vi "Get All Classes Properties and Methods.vi"(8 "error in":errorcluster) -> (0 "error out":errorcluster, 1 "Methods[]":T1(array[cluster]), 2 "Properties[]":T2(array[cluster]), 3 "All Classes Tree Sorted":T3(array[cluster]))   [LabVIEW 2023]
doc: "Gets all classes, properties, and methods available in LabVIEW. This is slow, as it also gets the R/W-ability, if scripting, private, etc. Best to do this once and cache the results."
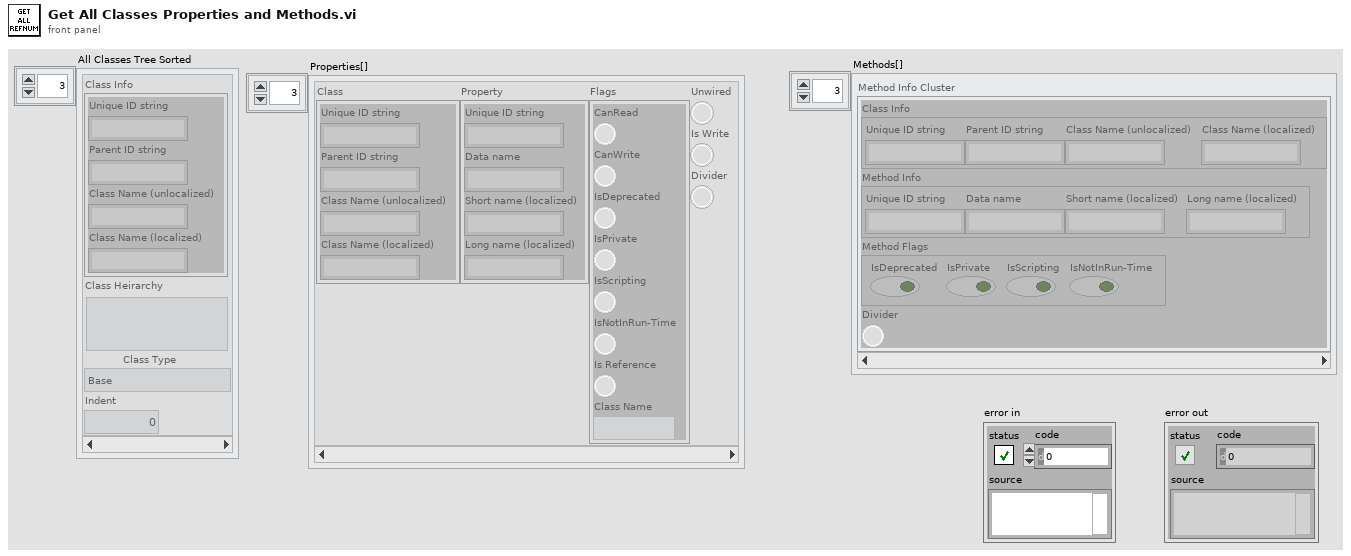
[diagram p1: front panel]
types:
  T1 = cluster{"Class Info":cluster{"Unique ID string":string, "Parent ID string":string, "Class Name (unlocalized)":string, "Class Name (localized)":string}, "Method Info":cluster{"Unique ID string":string, "Data name":string, "Short name (localized)":string, "Long name (localized)":string}, "Method Flags":cluster{"IsDeprecated":bool, "IsPrivate":bool, "IsScripting":bool, "IsNotInRun-Time":bool}, "Divider":bool}[]
  T2 = cluster{"Class":cluster{"Unique ID string":string, "Parent ID string":string, "Class Name (unlocalized)":string, "Class Name (localized)":string}, "Property":cluster{"Unique ID string":string, "Data name":string, "Short name (localized)":string, "Long name (localized)":string}, "Flags":cluster{"CanRead":bool, "CanWrite":bool, "IsDeprecated":bool, "IsPrivate":bool, "IsScripting":bool, "IsNotInRun-Time":bool, "Is Reference":bool, "Class Name":string}, "Divider":bool, "Is Write":bool, "Unwired":bool}[]
  T3 = cluster{"Class Info":cluster{"Unique ID string":string, "Parent ID string":string, "Class Name (unlocalized)":string, "Class Name (localized)":string}, "Class Heirarchy":string, "Class Type":enum16{"Unknown", "Base", "Scripting", "Private", "Deprecated", "None", "Divider"}, "Indent":u32}[]
  T4 = cluster{"Class Info":cluster{"Unique ID string":string, "Parent ID string":string, "Class Name (unlocalized)":string, "Class Name (localized)":string}, "Property Info":cluster{"Unique ID string":string, "Data name":string, "Short name (localized)":string, "Long name (localized)":string}, "Property Flags":cluster{"CanRead":bool, "CanWrite":bool, "IsDeprecated":bool, "IsPrivate":bool, "IsScripting":bool, "IsNotInRun-Time":bool, "Is Reference":bool, "Class Name":string}}[]
  T5 = cluster{"Class":cluster{"Unique ID string":string, "Parent ID string":string, "Class Name (unlocalized)":string, "Class Name (localized)":string}, "Property":cluster{"Unique ID string":string, "Data name":string, "Short name (localized)":string, "Long name (localized)":string}, "Flags":cluster{"CanRead":bool, "CanWrite":bool, "IsDeprecated":bool, "IsPrivate":bool, "IsScripting":bool, "IsNotInRun-Time":bool, "Is Reference":bool, "Class Name":string}, "Divider":bool, "Is Write":bool, "Unwired":bool}
  T6 = cluster{"Unique ID string":string, "Parent ID string":string, "Class Name (unlocalized)":string, "Class Name (localized)":string}
  T7 = cluster{"Unique ID string":string, "Data name":string, "Short name (localized)":string, "Long name (localized)":string}
  T8 = cluster{"CanRead":bool, "CanWrite":bool, "IsDeprecated":bool, "IsPrivate":bool, "IsScripting":bool, "IsNotInRun-Time":bool, "Is Reference":bool, "Class Name":string}
  T9 = cluster{"Class Info":cluster{"Unique ID string":string, "Parent ID string":string, "Class Name (unlocalized)":string, "Class Name (localized)":string}, "Method Info":cluster{"Unique ID string":string, "Data name":string, "Short name (localized)":string, "Long name (localized)":string}, "Method Flags":cluster{"IsDeprecated":bool, "IsPrivate":bool, "IsScripting":bool, "IsNotInRun-Time":bool}}[]
  T10 = cluster{"Class Info":cluster{"Unique ID string":string, "Parent ID string":string, "Class Name (unlocalized)":string, "Class Name (localized)":string}, "Method Info":cluster{"Unique ID string":string, "Data name":string, "Short name (localized)":string, "Long name (localized)":string}, "Method Flags":cluster{"IsDeprecated":bool, "IsPrivate":bool, "IsScripting":bool, "IsNotInRun-Time":bool}, "Divider":bool}
  T11 = cluster{"IsDeprecated":bool, "IsPrivate":bool, "IsScripting":bool, "IsNotInRun-Time":bool}
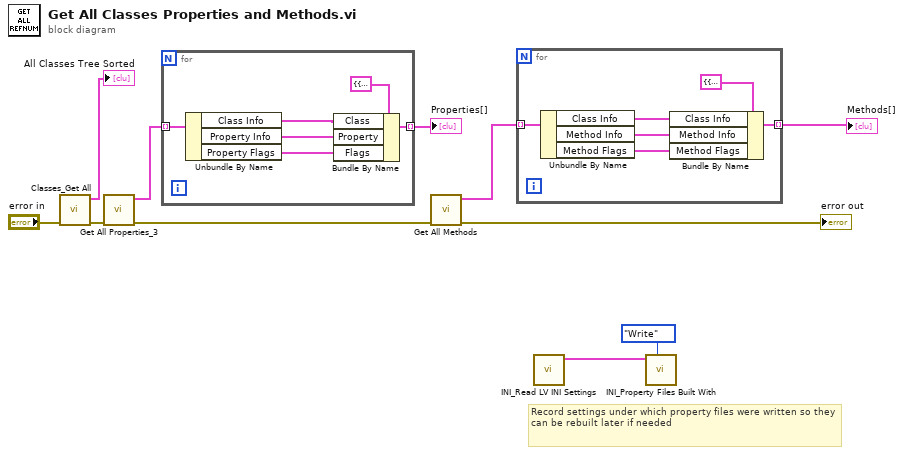
[diagram p0: block diagram]
diagram:
  # "Record settings under which property files were written so they can be rebuilt later if needed"
  n1 = call "Classes_Get All.vi"("error in"="error in") -> ("error out"=w10:errorcluster, "All Classes Tree Sorted"=→"All Classes Tree Sorted":T3)  [unwired: 9 in]
  n2 = call "Get All Properties_3.vi"("error in"=w10) -> ("error out"=w9:errorcluster, "Properties[]"=w5:T4)  [unwired: 9 in]
  n3 = for {
    tunnel: [w17] -> w6 mode=indexing
    tunnel: w5 -> [w15] mode=indexing
    n4 = Unbundle By Name(w15) -> ("Class Info"=w14:T6, "Property Info"=w13:T7, "Property Flags"=w12:T8)
    n5 = Bundle By Name(cluster=T5 {"Class"={"Unique ID string"="", "Parent ID string"="", "Class Name (unlocalized)"="", "Class Name (localized)"=""}, "Property"={"Unique ID string"="", "Data name"="", "Short name (localized)"="", "Long name (localized)"=""}, "Flags"={"CanRead"=FALSE, "CanWrite"=FALSE, "IsDeprecated"=FALSE, "IsPrivate"=FALSE, "IsScripting"=FALSE, "IsNotInRun-Time"=FALSE, "Is Reference"=FALSE, "Class Name"=""}, "Divider"=FALSE, "Is Write"=FALSE, "Unwired"=FALSE} ("Cluster"), "Class"=w14, "Property"=w13, "Flags"=w12) -> (w17:T5)
  }
  "Properties[]" <- w6
  n6 = call "Get All Methods.vi"("error in (no error)"=w9) -> ("error out"=→"error out":errorcluster, "Methods[]"=w4:T9)  [unwired: 9 in]
  n7 = for {
    tunnel: [w23] -> w3 mode=indexing
    tunnel: w4 -> [w21] mode=indexing
    n8 = Unbundle By Name(w21) -> ("Class Info"=w20:T6, "Method Info"=w19:T7, "Method Flags"=w18:T11)
    n9 = Bundle By Name(cluster=T10 {"Class Info"={"Unique ID string"="", "Parent ID string"="", "Class Name (unlocalized)"="", "Class Name (localized)"=""}, "Method Info"={"Unique ID string"="", "Data name"="", "Short name (localized)"="", "Long name (localized)"=""}, "Method Flags"={"IsDeprecated"=FALSE, "IsPrivate"=FALSE, "IsScripting"=FALSE, "IsNotInRun-Time"=FALSE}, "Divider"=FALSE} ("Method Info Cluster"), "Class Info"=w20, "Method Info"=w19, "Method Flags"=w18) -> (w23:T10)
  }
  "Methods[]" <- w3
  n10 = call "INI_Read LV INI Settings.vi"() -> ("LabVIEW INI Settings"=w1:cluster{"Scripting":bool, "Private":bool})  [unwired: 10 in, 1 out]
  n11 = call "INI_Property Files Built With.vi"("File Action"=enum16{"Read", "Write"}."Write", "Property Files Built With"=w1) -> ()  [unwired: 9 in, 1 out]
